vi "AudioTest.Get Audio Device List from PC.vi"() -> ()   [LabVIEW 2018]
panel:
  in  "Wave Volume":u32=60000
  in  "Speaker Volume":u32=60000 max=65535
  out "Success":bool
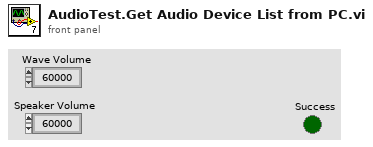
[diagram p1: front panel]
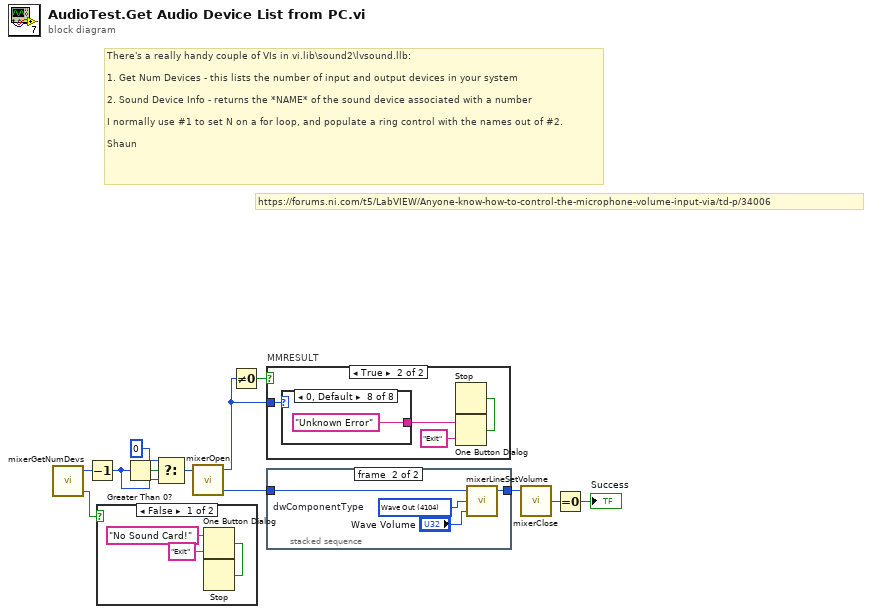
[diagram p0: block diagram]
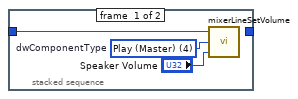
[diagram p2: hidden frame]
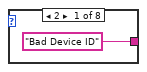
[diagram p4: hidden frame]
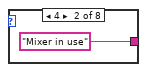
[diagram p5: hidden frame]
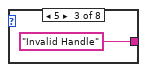
[diagram p6: hidden frame]
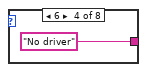
[diagram p7: hidden frame]
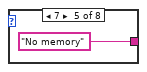
[diagram p8: hidden frame]
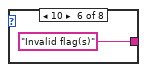
[diagram p9: hidden frame]
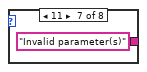
[diagram p10: hidden frame]
diagram:
  # "There's a really handy couple of VIs in vi.lib\\sound2\\lvsound.llb:\n\n1. Get Num Devices - this lists the number of input and output devices in your system\n\n2. Sound Device Info - returns the *NAME* of the sound device associated with a number\n\nI normally use #1 to set N on a for loop, and populate a ring control with the names out of #2.\n\nShaun"
  # "https://forums.ni.com/t5/LabVIEW/Anyone-know-how-to-control-the-microphone-volume-input-via/td-p/34006"
  n1 = call "mixerGetNumDevs.vi"() -> ("Found"=w12:bool, "Number of\nMixer Devices"=w5:u32)  [unwired: 4 in]
  n2 = Decrement(x=w5) -> (x-1=w9:u32)
  n3 = case shown="False" w12 {
    frame False {
      n4 = One Button Dialog(message="No Sound Card!", button name ("OK")="Exit") -> (true=w13:bool)
      n5 = Stop(stop? (T)=w13) -> ()
    }
    frame True {
      # "No Error"
    }
  }
  n6 = Greater Than 0?(x=w9) -> (x > 0?=w6:bool)
  n7 = Select(t=u32 0 ("y"), s=w6, f=w9) -> (s? t:f=w8:u32)
  n8 = call "mixerOpen.vi"("uMxId"=w8) -> ("phmx"=w4:u32, "MMRESULT"=w10:u32)  [unwired: 3 in]
  n9 = Not Equal To 0?(x=w10) -> (x != 0?=w11:bool)
  n10 = case "MMRESULT" shown="True" w11 {
    tunnel: w10 -> [_ w19]
    frame False {
      # "No Error"
    }
    frame True {
      n11 = case shown="0, Default" w19 {
        tunnel: ["Bad Device ID" ("message") "Mixer in use" ("message") "Invalid Handle" ("message") "No driver" ("message") "No memory" ("message") "Invalid flag(s)" ("message") "Invalid parameter(s)" ("message") "Unknown Error" ("message")] -> w17
        frame 2 {
        }
        frame 4 {
        }
        frame 5 {
        }
        frame 6 {
        }
        frame 7 {
        }
        frame 10 {
        }
        frame 11 {
        }
        frame 0, Default {
        }
      }
      n12 = One Button Dialog(message=w17, button name ("OK")="Exit") -> (true=w16:bool)
      n13 = Stop(stop? (T)=w16) -> ()
    }
  }
  n14 = stacked-sequence {
    tunnel: w4 -> [w29 w34]
    tunnel: [_ w31] -> w1
    frame #0 {
      w28 = u32 4 items=["Play (Master)"=4, "CD Audio"=4112, "Line In"=4098, "Microphone In"=4099, "PC Speaker"=4103, "Auxiliary In"=4105, "TAD In"=4102, "Wave Out"=4104, "MIDI"=4100, "CD Digital"=4097]  # dwComponentType
      n15 = call "mixerLineSetVolume.vi"("Volume"="Speaker Volume", "dwComponentType"=w28, "hmxobj"=w29) -> ()  [unwired: 1 in, 2 out]
    }
    frame #1 {
      w33 = u32 4104 items=["Play (Master)"=4, "CD Audio"=4112, "Line In"=4098, "Microphone In"=4099, "PC Speaker"=4103, "Auxiliary In"=4105, "TAD In"=4102, "Wave Out"=4104, "MIDI"=4100, "CD Digital"=4097]  # dwComponentType
      n16 = call "mixerLineSetVolume.vi"("Volume"="Wave Volume", "dwComponentType"=w33, "hmxobj"=w34) -> ("hmxobj Out"=w31:u32)  [unwired: 1 in, 1 out]
    }
  }
  n17 = call "mixerClose.vi"("hmx"=w1) -> ("MMRESULT"=w2:u32)  [unwired: 4 in]
  n18 = Equal To 0?(x=w2) -> (x = 0?=→"Success":bool)
